vi "isCalZeroable.vi"(8 "Inst type":T1, 11 "Calib File":path) -> (2 "Zeroable?":bool)   [LabVIEW 2022 SP3]
uses:
  Controls/Inst_type.ctl
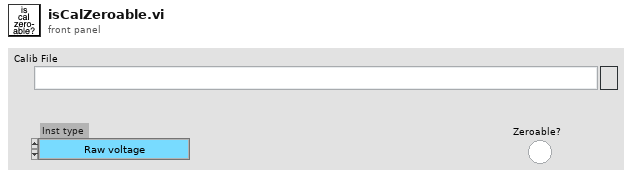
[diagram p1: front panel]
types:
  T1 = typedef "Inst_type.ctl" = enum16{"Raw voltage", "Raw with zero offsetting", "Propeller anemometer", "Pressure Transducer", "Pitot-static tube", "Hot wire", "Cross wire 1", "Cross wire 2", "Generic Linear", "Generic Polynomial", "Generic BackPoly", "Fast FID", "Thermocouple", "Cold wire", "Pulsed Wire", "LDA Vel", "LDA Tran time", "LDA Arr time", "Microphone"}
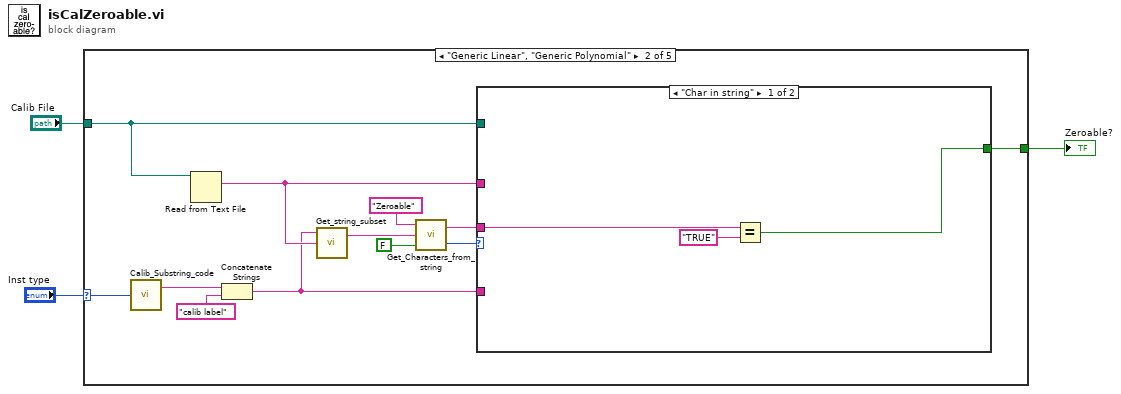
[diagram p0: block diagram]
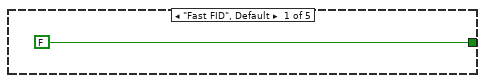
[diagram p2: hidden frame]
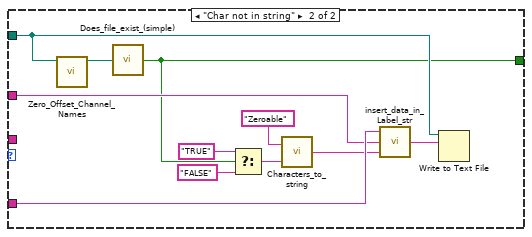
[diagram p3: hidden frame]
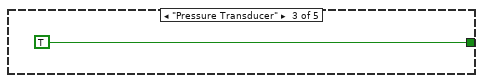
[diagram p4: hidden frame]
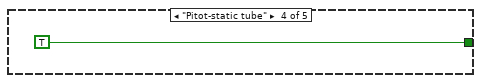
[diagram p5: hidden frame]
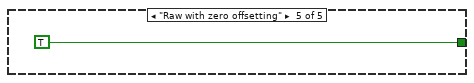
[diagram p6: hidden frame]
diagram:
  n1 = case shown="\"Generic Linear\", \"Generic Polynomial\"" "Inst type" {
    selector: "Inst type" -> [_ w15 _ _ _]
    tunnel: [FALSE ("exists?") w16 TRUE ("exists?") TRUE ("exists?") TRUE ("exists?")] -> w2
    tunnel: "Calib File" -> [_ w14 _ _ _]
    frame "Fast FID", Default {
    }
    frame "Generic Linear", "Generic Polynomial" {
      n2 = call "Calib_Substring_code.vi"("Inst type"=w15) -> ("Substring Type"=w8:string)  [unwired: 1 out]
      n3 = Read from Text File(file (use dialog)=w14) -> (text=w12:string)  [unwired: 3 in, 3 out]
      n4 = Concatenate Strings(w8, "calib label") -> (w11:string)
      n5 = call "Get_string_subset.vi"("String to split"=w12, "File Label"=w11) -> ("Output string"=w5:string)  [unwired: 2 in, 1 out]
      n6 = call "Get_Characters_from_string.vi"("Show Dialog?"=FALSE, "Input string"=w5, "Variable name"="Zeroable") -> ("Status"=w13:enum16{"Char in string", "Char not in string"}, "Value"=w10:string)
      n7 = case shown="\"Char in string\"" w13 {
        tunnel: w14 -> [_ w21]
        tunnel: w11 -> [_ w25]
        tunnel: w12 -> [_ w24]
        tunnel: w10 -> [w19 _]
        tunnel: [w17 w20] -> w16
        frame "Char in string" {
          n8 = Equal?(x=w19, y="TRUE") -> (x = y?=w17:bool)
        }
        frame "Char not in string" {
          n9 = call "Zero_Offset_Channel_Names.vi"("Calib Filename"=w21) -> ("Zero Filename"=w30:path)  [unwired: 3 in, 3 out]
          n10 = call "Does_file_exist_(simple).vi"("Pathname"=w30) -> ("exists?"=w20:bool)
          n11 = Select(t="TRUE", s=w20, f="FALSE") -> (s? t:f=w26:string)
          n12 = call "Characters_to_string.vi"("Characters to write"=w26, "Label for characters"="Zeroable") -> ("Output string"=w23:string)  [unwired: 1 in]
          n13 = call "insert_data_in_Label_str.vi"("dataToInsert"=w23, "Input string"=w24, "label name"=w25) -> ("Appended string"=w22:string)
          n14 = Write to Text File(file (use dialog)=w21, text=w22) -> ()  [unwired: 2 in, 3 out]
        }
      }
    }
    frame "Pressure Transducer" {
    }
    frame "Pitot-static tube" {
    }
    frame "Raw with zero offsetting" {
    }
  }
  "Zeroable?" <- w2
